vi "Calculos_ventana.vi"(4 "Distancias generales":dbl, 5 "Longitud de ventana":dbl, 6 "Velocidad de ejes":dbl, 7 "Puntos":sgl, 9 "Frecuencia de muestreo":dbl, 10 "Loop Iteration":i32, 11 "Distancias acelerometros":dbl[](array[numeric])) -> (1 "Punto inicial de la ventana":dbl, 2 "Valores truncados a la baja":dbl, 3 "Offset":dbl)   [LabVIEW 2015]
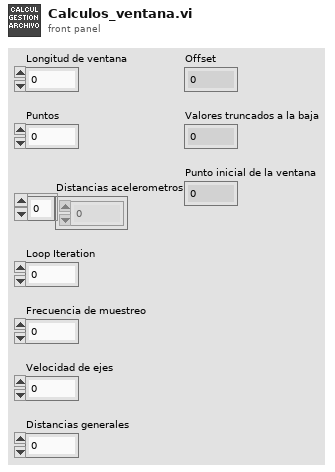
[diagram p1: front panel]
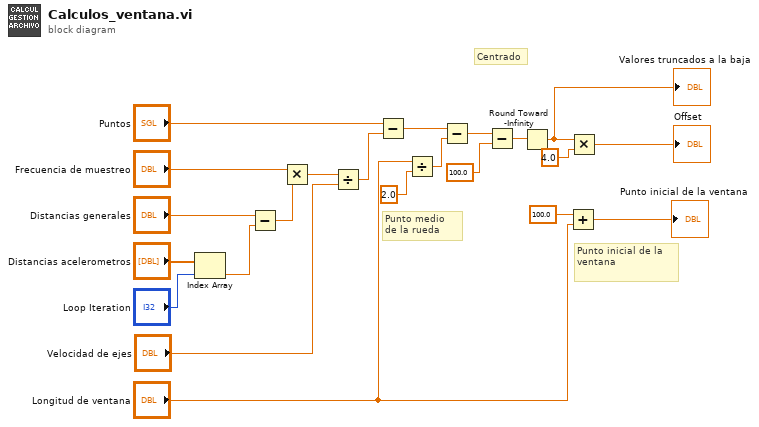
[diagram p0: block diagram]
diagram:
  # "Centrado"
  # "Punto inicial de la \nventana"
  # "Punto medio\nde la rueda"
  n1 = Index Array(array="Distancias acelerometros", index="Loop Iteration") -> (element=w18:dbl)
  n2 = Subtract(x="Distancias generales", y=w18) -> (x-y=w9:dbl)
  n3 = Multiply(x="Frecuencia de muestreo", y=w9) -> (x*y=w7:dbl)
  n4 = Divide(x=w7, y="Velocidad de ejes") -> (x/y=w8:dbl)
  n5 = Subtract(x="Puntos", y=w8) -> (x-y=w12:dbl)
  n6 = Divide(x="Longitud de ventana", y=2.0) -> (x/y=w11:dbl)
  n7 = Subtract(x=w12, y=w11) -> (x-y=w16:dbl)
  n8 = Subtract(x=w16, y=100.0 ("x")) -> (x-y=w13:dbl)
  n9 = Round Toward -Infinity(1:w13) -> (0:w21:dbl)
  "Valores truncados a la baja" <- w21
  n10 = Add(x=100.0, y="Longitud de ventana") -> (x+y=→"Punto inicial de la ventana":dbl)
  n11 = Multiply(x=w21, y=4.0) -> (x*y=→"Offset":dbl)
